vi "All X[i] = X[0] [DBL].vi"(1 "Tolerance (1E-6)":dbl=1e-06, 7 "X":dbl[](array[numeric]) format="%#_9g") -> (8 "All Identical?":bool)   [LabVIEW 2021, in "Comparison.lvlib"]
doc: "Checks whether all elements of the array are identical within the provided tolerance."
uses:
  Comparison.lvlib
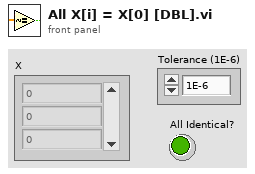
[diagram p1: front panel]
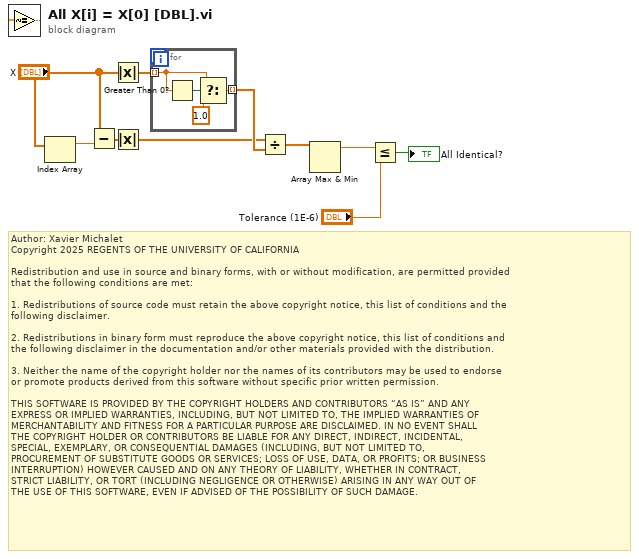
[diagram p0: block diagram]
diagram:
  # "Author: Xavier Michalet\nCopyright 2025 REGENTS OF THE UNIVERSITY OF CALIFORNIA\n\nRedistribution and use in source and binary forms, with or without modification, are permitted provided\nthat the following conditions are met:\n\n1. Redistributions of source code must retain the above copyright notice, this list of conditions and the\nfollowing disclaimer.\n\n2. Redistributions in binary form must reproduce the above copyright notice, this list of conditions and\nthe following disclaimer in the documentation and/or other materials provided with the distribution.\n\n3. Neither the name of the copyright holder nor the names of its contributors may be used to endorse \nor promote products derived from this software without specific prior written permission.\n\nTHIS SOFTWARE IS PROVIDED BY THE COPYRIGHT HOLDERS AND CONTRIBUTORS “AS IS” AND ANY \nEXPRESS OR IMPLIED WARRANTIES, INCLUDING, BUT NOT LIMITED TO, THE IMPLIED WARRANTIES OF\nMERCHANTABILITY AND FITNESS FOR A PARTICULAR PURPOSE ARE DISCLAIMED. IN NO EVENT SHALL\nTHE COPYRIGHT HOLDER OR CONTRIBUTORS BE LIABLE FOR ANY DIRECT, INDIRECT, INCIDENTAL, \nSPECIAL, EXEMPLARY, OR CONSEQUENTIAL DAMAGES (INCLUDING, BUT NOT LIMITED TO, \nPROCUREMENT OF SUBSTITUTE GOODS OR SERVICES; LOSS OF USE, DATA, OR PROFITS; OR BUSINESS\nINTERRUPTION) HOWEVER CAUSED AND ON ANY THEORY OF LIABILITY, WHETHER IN CONTRACT, \nSTRICT LIABILITY, OR TORT (INCLUDING NEGLIGENCE OR OTHERWISE) ARISING IN ANY WAY OUT OF\nTHE USE OF THIS SOFTWARE, EVEN IF ADVISED OF THE POSSIBILITY OF SUCH DAMAGE."
  n1 = Index Array(array="X") -> (element=w1:dbl)  [unwired: 1 in]
  n2 = Subtract(x="X", y=w1) -> (x-y=w8:dbl[])
  n3 = Absolute Value(x="X") -> (abs(x)=w7:dbl[])
  n4 = Absolute Value(x=w8) -> (abs(x)=w5:dbl[])
  n5 = for {
    tunnel: w7 -> [w13] mode=indexing
    tunnel: [w11] -> w6 mode=indexing
    n6 = Greater Than 0?(x=w13) -> (x > 0?=w14:bool)
    n7 = Select(t=w13, s=w14, f=1.0) -> (s? t:f=w11:dbl)
  }
  n8 = Divide(x=w5, y=w6) -> (x/y=w4:dbl[])
  n9 = Array Max & Min(array=w4) -> (max value=w10:dbl)  [unwired: 3 out]
  n10 = Less Or Equal?(x=w10, y="Tolerance (1E-6)") -> (x <= y?=→"All Identical?":bool)
